vi "LS330_OpenLog.vi"(9 "Prefix":string="TempFile_", 11 "Log Location":path) -> (0 "error out":errorcluster, 1 "file or folder exists?":bool, 3 "File RefOut":refnum<file>)   [LabVIEW 2021]
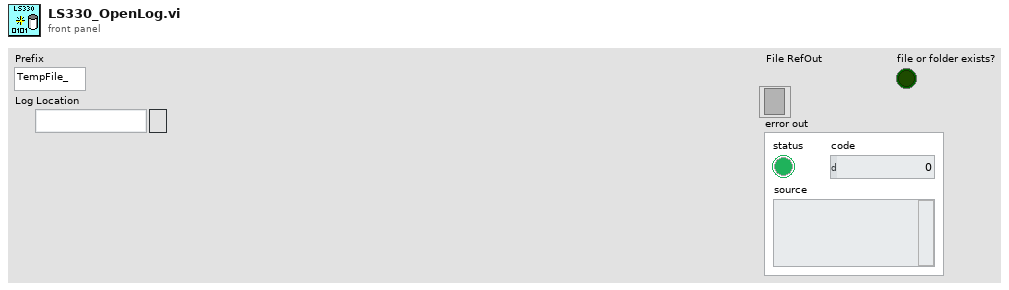
[diagram p1: front panel]
types:
  T1 = enum16{"open", "replace", "create", "open or create", "replace or create", "replace or create with confirmation"}
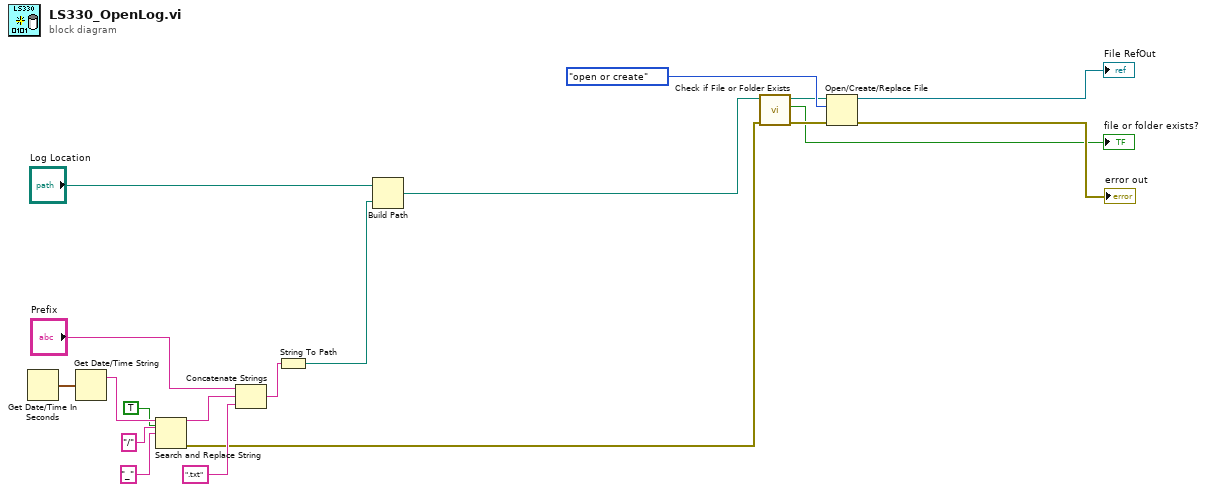
[diagram p0: block diagram]
diagram:
  n1 = Get Date/Time In Seconds() -> (seconds since 1Jan1904=w19:timestamp)
  n2 = Get Date/Time String(seconds (now)=w19) -> (date string=w18:string)  [unwired: 2 in, 1 out]
  n3 = Search and Replace String(replace all?=TRUE ("replace all? (F)"), input string=w18, search string="/", replace string="_" ("replace string (\"\")")) -> (result string=w14:string, error out=w2:errorcluster)  [unwired: 4 in, 2 out]
  n4 = Concatenate Strings("Prefix", w14, ".txt" ("string")) -> (w13:string)
  n5 = String To Path(string=w13) -> (path=w4:path)
  n6 = Build Path(base path="Log Location", name or relative path=w4) -> (appended path=w3:path)
  n7 = call <vilib>:"Check if File or Folder Exists.vi"("error in (no error)"=w2, "path"=w3) -> ("error out"=w7:errorcluster, "file or folder exists?"=→"file or folder exists?":bool, "dup path"=w8:path)  [unwired: 7 in]
  n8 = Open/Create/Replace File(file path (use dialog)=w8, error in=w7, operation (0:open)=T1."open or create") -> (refnum out=→"File RefOut":refnum<file>, error out=→"error out":errorcluster)  [unwired: 3 in, 1 out]
